vi "Write Text.vi"(8 "error in (no error)":errorcluster, 10 "Text":string, 11 "Tag_LVOOP.lvclass in":refnum<class "Tree Tag Class.lvclass">) -> (0 "error out":errorcluster, 3 "Tag_LVOOP.lvclass out":refnum<class "Tree Tag Class.lvclass">)   [LabVIEW 2012, in "Tree Tools.lvlib" / "Tree Tag Class.lvclass"]
uses:
  Tree Tag Class.lvclass
  Tree Tag Class.lvclass/Tree Tag Class.ctl
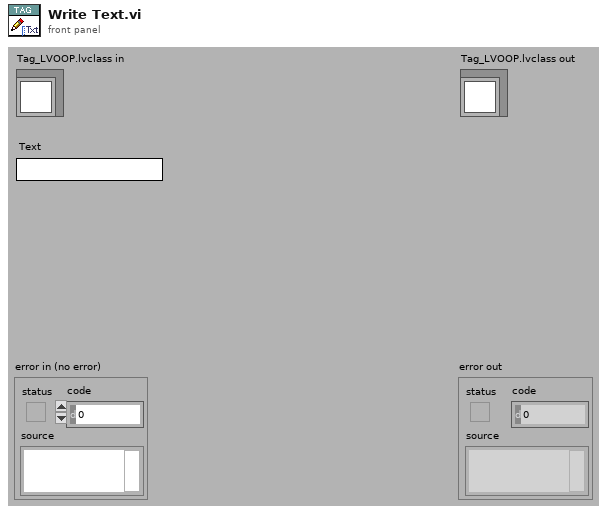
[diagram p1: front panel]
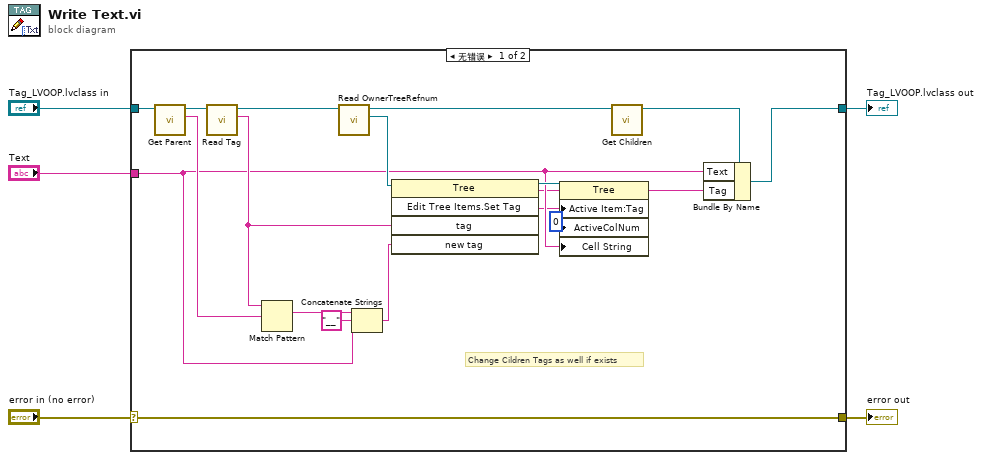
[diagram p0: block diagram]
diagram:
  n1 = case shown="无错误" "error in (no error)" {
    selector: "error in (no error)" -> [w22 w23]
    tunnel: [w22 w23] -> w4
    tunnel: [w21 w24] -> w2
    tunnel: "Tag_LVOOP.lvclass in" -> [w20 w24]
    tunnel: "Text" -> [w8 _]
    frame No Error {
      # "Change Cildren Tags as well if exists"
      n2 = call-dynamic "Get Parent.vi"("Tag_LVOOP in"=w20) -> ("Parent Tag string"=w13:string, "Tag_LVOOP out"=w19:refnum<class "Tree Tag Class.lvclass">)  [unwired: 1 in, 8 out]
      n3 = call-dynamic "Read Tag.vi"("Tag_LVOOP.lvclass in"=w19) -> ("Tag"=w14:string, "Tag_LVOOP.lvclass out"=w18:refnum<class "Tree Tag Class.lvclass">)  [unwired: 1 in, 8 out]
      n4 = Match Pattern(string=w14, regular expression=w13) -> (match substring=w12:string)  [unwired: 4 out]
      n5 = call-dynamic "Read OwnerTreeRefnum.vi"("Tag_LVOOP.lvclass in"=w18) -> ("Owner (Tree Refnum)"=w17:refnum<vi>, "Tag_LVOOP.lvclass out"=w11:refnum<class "Tree Tag Class.lvclass">)  [unwired: 1 in, 8 out]
      n6 = Concatenate Strings(w12, "__" ("string"), w8) -> (w7:string)
      n7 = invoke class="Tree" method="Edit Tree Items.Set Tag"(reference=w17, "tag"=w14, "new tag"=w7) -> (reference out=w16:refnum<vi>, "Edit Tree Items:Set Tag"=w6:string)  [unwired: 2 in, 3 out]
      n8 = property class="Tree"(reference=w16, "Active Item:Tag"=w6, "ActiveColNum"=0 ("Active Cell:Active Column Number"), "Cell String"=w8) -> ()  [unwired: 1 in, 2 out]
      n9 = call-dynamic "Get Children.vi"("Tag_LVOOP in"=w11) -> ("Tag_LVOOP out"=w10:refnum<class "Tree Tag Class.lvclass">)  [unwired: 1 in, 9 out]
      n10 = Bundle By Name(cluster=w10, "Text"=w8, "Tag"=w6) -> (w21:refnum<class "Tree Tag Class.lvclass">)
    }
    frame Error {
    }
  }
  "error out" <- w4
  "Tag_LVOOP.lvclass out" <- w2
